vi "Read FW Version.vi"(8 "error in (no error)":errorcluster, 11 "Data in":refnum<class "Data.lvclass">) -> (0 "error out":errorcluster, 2 "FW Version":string="0.0.0", 3 "Data out":refnum<class "Data.lvclass">)   [LabVIEW 2018, in "HW Interaction.lvlib" / "Data.lvclass"]
uses:
  Data.lvclass
  Data.lvclass/Data.ctl
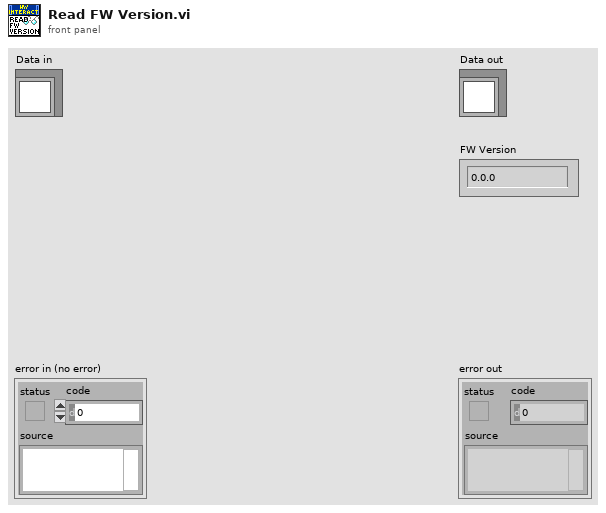
[diagram p1: front panel]
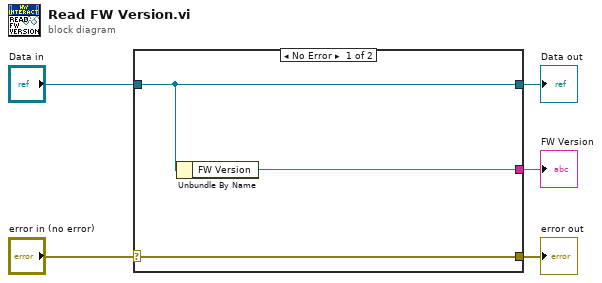
[diagram p0: block diagram]
diagram:
  n1 = case shown="No Error" "error in (no error)" {
    selector: "error in (no error)" -> [w8 w9]
    tunnel: [w8 w9] -> w4
    tunnel: [w7 w10] -> w2
    tunnel: "Data in" -> [w7 w10]
    tunnel: [w6 _] -> w1
    frame No Error {
      n2 = Unbundle By Name(w7) -> ("FW Version"=w6:string)
    }
    frame Error {
    }
  }
  "error out" <- w4
  "Data out" <- w2
  "FW Version" <- w1
